vi "To Tree Data.vi"   [LabVIEW 2020, in "NI_VIAnCFGDataStructure.lvlib" / "Tree.lvclass"]
doc: "Polymorphic instance of the To Tree Data method. Select the appropraite instance to work with or allow this method to adapt automatically."
uses:
  <vilib>/addons/analyzer/VIAnCFGDataStructure/Tree Manager/Tree.lvclass
  <vilib>/addons/analyzer/VIAnCFGDataStructure/Data Types/Bool/Bool.lvclass
  <vilib>/addons/analyzer/VIAnCFGDataStructure/Data Types/Int/Int.lvclass
  <vilib>/addons/analyzer/VIAnCFGDataStructure/Data Types/Float/Flt.lvclass
  <vilib>/addons/analyzer/VIAnCFGDataStructure/Data Types/String/String.lvclass
  <vilib>/addons/analyzer/VIAnCFGDataStructure/Data Types/Path/Path.lvclass
  <vilib>/addons/analyzer/VIAnCFGDataStructure/Data Types/String Array/1D String.lvclass
  <vilib>/addons/analyzer/VIAnCFGDataStructure/Data Types/Bool Array/1D Bool.lvclass
  <vilib>/addons/analyzer/VIAnCFGDataStructure/Data Types/Flt Array/1D Flt.lvclass
  <vilib>/addons/analyzer/VIAnCFGDataStructure/Data Types/Int Array/1D Int.lvclass
  <vilib>/addons/analyzer/VIAnCFGDataStructure/Data Types/Path Array/1D Path.lvclass
  <vilib>/addons/analyzer/VIAnCFGDataStructure/Data Types/2D Bool/2D Bool.lvclass
  <vilib>/addons/analyzer/VIAnCFGDataStructure/Data Types/2D Int/2D Int.lvclass
  <vilib>/addons/analyzer/VIAnCFGDataStructure/Data Types/2D Flt/2D Flt.lvclass
  <vilib>/addons/analyzer/VIAnCFGDataStructure/Data Types/2D Path/2D Path.lvclass
  <vilib>/addons/analyzer/VIAnCFGDataStructure/Data Types/2D String/2D String.lvclass
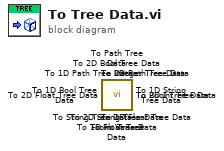
[diagram p0: block diagram]
diagram:
  n1 = call <vilib>:"To 2D String Tree Data.vi"() -> ()  [unwired: 11 in, 1 out]
  n2 = call <vilib>:"To 2D Path Tree Data.vi"() -> ()  [unwired: 11 in, 1 out]
  n3 = call <vilib>:"To 2D Float Tree Data.vi"() -> ()  [unwired: 11 in, 1 out]
  n4 = call <vilib>:"To 2D Int Tree Data.vi"() -> ()  [unwired: 11 in, 1 out]
  n5 = call <vilib>:"From Variant.vi"() -> ()  [unwired: 10 in, 2 out]
  n6 = call <vilib>:"To 2D Bool Tree Data.vi"() -> ()  [unwired: 11 in, 1 out]
  n7 = call <vilib>:"To 1D Path Tree Data.vi"() -> ()  [unwired: 11 in, 1 out]
  n8 = call <vilib>:"To 1D Int Tree Data.vi"() -> ()  [unwired: 11 in, 1 out]
  n9 = call <vilib>:"To 1D Float Tree Data.vi"() -> ()  [unwired: 11 in, 1 out]
  n10 = call <vilib>:"To 1D Bool Tree Data.vi"() -> ()  [unwired: 11 in, 1 out]
  n11 = call <vilib>:"To 1D String Tree Data.vi"() -> ()  [unwired: 11 in, 1 out]
  n12 = call <vilib>:"To Path Tree Data.vi"() -> ()  [unwired: 11 in, 1 out]
  n13 = call <vilib>:"To String Tree Data.vi"() -> ()  [unwired: 11 in, 1 out]
  n14 = call <vilib>:"To Float Tree Data.vi"() -> ()  [unwired: 11 in, 1 out]
  n15 = call <vilib>:"To Integer Tree Data.vi"() -> ()  [unwired: 11 in, 1 out]
  n16 = call <vilib>:"To Bool Tree Data.vi"() -> ()  [unwired: 11 in, 1 out]
